vi "CompareZProfile2.vi"(5 "Z profile":dbl[](array[numeric])=[136.78057938360504, 136.0261652116635, 136.02991437413465, 127.00664231648236, 122.29049463775536, 113.645207456899, 109.8856960808644, 104.76567514371389, 100.83691644163049, 97.71438212515365, 93.93238486999432, 90.08654473167638, 87.00841340233623, 84.35416666666667, 81.7528515593838, 79.6393412331386, 83.05002287132794, 85.13533535994708, 91.11477171457702, 98.5078614332252, 103.77404656553082, 105.17571186727207, 109.49616358691677, 109.23224687693282, 112.95297246100046, 117.20435850121594, 115.42078946409929, 112.54404430067521, 102.6815824186669, 91.80857555867811, 81.43765852235101, 76.84419557315564, 77.3156658575995, 83.36916637000127, 89.63776385905682, 93.40653392326749, 107.04734731706081, 119.8811021895823, 151.17114676843892, 187.80852396310843, 214.26554708781225, 232.30872499497298, 224.32904818821265, 191.3640629515997, 147.3785829578186, 102.59016510146526, 80.02115124526546, 81.1632766895408, 95.07169339561545, 120.10465998090932, 137.718697100722, 143.98076644746772, 147.53366304165087, 141.65846157484788, 134.07428104411483, 129.81679576307346, 126.37067033940068, 121.24591602303097, 125.47090035098631, 122.74778342807349, 123.40827458303652, 123.34074109763333, 123.50642201559259, 120.7960259846455, 122.26527340257906] format="%.2f", 6 "Z LUT":dbl[][](array[numeric])=[[137.0, 137.0, 137.0, 130.0, 125.0, 119.0, 113.0, 108.0, 109.0, 114.0, 121.0, 127.0, 133.0, 139.0, 146.0, 153.0, 156.0, 151.0, 132.0, 100.0, 66.0, 46.0, 50.0, 72.0, 99.0, 119.0, 132.0, 138.0, 142.0, 146.0, 148.0, 149.0, 147.0, 143.0, 138.0, 133.0, 129.0, 128.0, 129.0, 130.0, 132.0, 134.0, 133.0, 132.0, 131.0, 130.0, 129.0, 129.0, 130.0, 130.0, 130.0, 130.0, 131.0, 131.0, 131.0, 131.0, 131.0, 131.0, 131.0, 131.0, 131.0, 131.0, 131.0, 131.0, 132.0], [135.0, 133.0, 130.0, 129.0, 130.0, 128.0, 119.0, 109.0, 101.0, 100.0, 104.0, 111.0, 119.0, 126.0, 134.0, 146.0, 162.0, 171.0, 164.0, 133.0, 88.0, 53.0, 42.0, 55.0, 80.0, 103.0, 124.0, 139.0, 151.0, 159.0, 160.0, 156.0, 150.0, 142.0, 135.0, 130.0, 128.0, 127.0, 130.0, 132.0, 132.0, 132.0, 131.0, 130.0, 130.0, 130.0, 130.0, 130.0, 131.0, 131.0, 129.0, 130.0, 131.0, 131.0, 132.0, 129.0, 131.0, 131.0, 132.0, 133.0, 133.0, 131.0, 131.0, 130.0, 132.0], [129.0, 128.0, 127.0, 127.0, 130.0, 129.0, 123.0, 114.0, 106.0, 98.0, 94.0, 95.0, 99.0, 107.0, 119.0, 142.0, 167.0, 186.0, 189.0, 163.0, 113.0, 63.0, 36.0, 37.0, 60.0, 87.0, 116.0, 139.0, 158.0, 168.0, 168.0, 161.0, 150.0, 141.0, 133.0, 129.0, 131.0, 130.0, 131.0, 132.0, 132.0, 132.0, 132.0, 131.0, 131.0, 130.0, 129.0, 130.0, 131.0, 130.0, 131.0, 131.0, 130.0, 130.0, 131.0, 130.0, 131.0, 132.0, 130.0, 131.0, 131.0, 131.0, 131.0, 131.0, 131.0], [129.0, 125.0, 125.0, 124.0, 127.0, 127.0, 124.0, 119.0, 111.0, 100.0, 91.0, 85.0, 85.0, 91.0, 103.0, 126.0, 159.0, 188.0, 200.0, 185.0, 140.0, 85.0, 43.0, 30.0, 42.0, 69.0, 103.0, 137.0, 163.0, 176.0, 176.0, 166.0, 154.0, 143.0, 136.0, 132.0, 131.0, 131.0, 131.0, 132.0, 132.0, 131.0, 132.0, 131.0, 131.0, 130.0, 130.0, 131.0, 130.0, 130.0, 130.0, 131.0, 130.0, 129.0, 129.0, 131.0, 130.0, 131.0, 130.0, 130.0, 130.0, 131.0, 131.0, 132.0, 132.0], [131.0, 126.0, 123.0, 121.0, 121.0, 123.0, 123.0, 120.0, 114.0, 104.0, 94.0, 85.0, 81.0, 82.0, 89.0, 106.0, 137.0, 174.0, 198.0, 197.0, 165.0, 115.0, 67.0, 39.0, 33.0, 49.0, 84.0, 126.0, 162.0, 181.0, 184.0, 175.0, 162.0, 150.0, 141.0, 135.0, 130.0, 129.0, 130.0, 132.0, 131.0, 130.0, 130.0, 131.0, 130.0, 131.0, 131.0, 132.0, 131.0, 130.0, 129.0, 130.0, 130.0, 130.0, 129.0, 130.0, 130.0, 131.0, 130.0, 131.0, 131.0, 131.0, 131.0, 131.0, 132.0], [132.0, 128.0, 122.0, 119.0, 117.0, 117.0, 118.0, 116.0, 112.0, 107.0, 100.0, 92.0, 87.0, 82.0, 82.0, 90.0, 113.0, 148.0, 179.0, 193.0, 181.0, 146.0, 102.0, 62.0, 37.0, 35.0, 61.0, 108.0, 152.0, 181.0, 190.0, 186.0, 174.0, 162.0, 148.0, 138.0, 130.0, 127.0, 127.0, 129.0, 130.0, 129.0, 129.0, 130.0, 129.0, 130.0, 131.0, 132.0, 132.0, 131.0, 130.0, 130.0, 131.0, 131.0, 131.0, 130.0, 130.0, 131.0, 132.0, 132.0, 132.0, 131.0, 131.0, 131.0, 132.0], [132.0, 128.0, 124.0, 120.0, 117.0, 114.0, 112.0, 111.0, 108.0, 106.0, 103.0, 99.0, 95.0, 90.0, 84.0, 84.0, 94.0, 120.0, 149.0, 174.0, 181.0, 168.0, 137.0, 95.0, 54.0, 33.0, 43.0, 83.0, 131.0, 169.0, 192.0, 197.0, 190.0, 176.0, 159.0, 144.0, 134.0, 127.0, 125.0, 125.0, 127.0, 128.0, 129.0, 130.0, 129.0, 130.0, 131.0, 132.0, 131.0, 131.0, 130.0, 130.0, 131.0, 131.0, 132.0, 131.0, 130.0, 131.0, 133.0, 133.0, 132.0, 131.0, 130.0, 131.0, 132.0], [131.0, 127.0, 125.0, 124.0, 119.0, 114.0, 110.0, 108.0, 105.0, 103.0, 101.0, 101.0, 100.0, 98.0, 94.0, 89.0, 87.0, 100.0, 119.0, 144.0, 164.0, 171.0, 161.0, 128.0, 82.0, 45.0, 34.0, 58.0, 102.0, 147.0, 185.0, 203.0, 205.0, 192.0, 174.0, 155.0, 139.0, 130.0, 124.0, 123.0, 125.0, 127.0, 128.0, 130.0, 130.0, 131.0, 132.0, 131.0, 130.0, 131.0, 130.0, 130.0, 129.0, 130.0, 131.0, 131.0, 131.0, 131.0, 132.0, 132.0, 132.0, 131.0, 132.0, 131.0, 132.0], [129.0, 125.0, 125.0, 125.0, 122.0, 117.0, 111.0, 108.0, 104.0, 101.0, 98.0, 98.0, 99.0, 102.0, 101.0, 98.0, 93.0, 94.0, 101.0, 115.0, 136.0, 156.0, 165.0, 151.0, 115.0, 70.0, 40.0, 42.0, 70.0, 116.0, 166.0, 200.0, 216.0, 209.0, 194.0, 172.0, 151.0, 134.0, 125.0, 122.0, 124.0, 126.0, 127.0, 129.0, 132.0, 132.0, 133.0, 131.0, 129.0, 131.0, 130.0, 130.0, 128.0, 129.0, 130.0, 130.0, 131.0, 131.0, 132.0, 131.0, 131.0, 130.0, 132.0, 131.0, 132.0], [129.0, 123.0, 125.0, 123.0, 122.0, 119.0, 114.0, 110.0, 105.0, 102.0, 97.0, 95.0, 94.0, 98.0, 102.0, 105.0, 102.0, 100.0, 97.0, 99.0, 111.0, 131.0, 151.0, 155.0, 138.0, 102.0, 61.0, 40.0, 46.0, 81.0, 135.0, 184.0, 216.0, 223.0, 216.0, 194.0, 169.0, 143.0, 128.0, 121.0, 121.0, 123.0, 126.0, 129.0, 133.0, 133.0, 134.0, 132.0, 131.0, 131.0, 130.0, 130.0, 129.0, 129.0, 129.0, 129.0, 130.0, 130.0, 131.0, 130.0, 129.0, 129.0, 131.0, 130.0, 133.0], [132.0, 123.0, 124.0, 122.0, 121.0, 119.0, 116.0, 112.0, 107.0, 103.0, 98.0, 93.0, 91.0, 91.0, 96.0, 103.0, 107.0, 109.0, 105.0, 100.0, 100.0, 109.0, 127.0, 143.0, 144.0, 126.0, 91.0, 56.0, 39.0, 53.0, 98.0, 153.0, 202.0, 227.0, 234.0, 217.0, 193.0, 161.0, 136.0, 121.0, 116.0, 118.0, 123.0, 128.0, 132.0, 133.0, 134.0, 133.0, 133.0, 131.0, 130.0, 130.0, 129.0, 130.0, 129.0, 129.0, 130.0, 129.0, 130.0, 129.0, 129.0, 129.0, 129.0, 130.0, 134.0], [135.0, 124.0, 125.0, 121.0, 119.0, 117.0, 114.0, 111.0, 107.0, 103.0, 98.0, 94.0, 90.0, 86.0, 88.0, 94.0, 104.0, 111.0, 114.0, 110.0, 105.0, 102.0, 108.0, 121.0, 132.0, 133.0, 115.0, 83.0, 52.0, 43.0, 65.0, 114.0, 172.0, 216.0, 240.0, 237.0, 219.0, 187.0, 153.0, 128.0, 114.0, 111.0, 116.0, 124.0, 129.0, 132.0, 134.0, 134.0, 133.0, 132.0, 131.0, 130.0, 130.0, 130.0, 130.0, 130.0, 131.0, 130.0, 130.0, 129.0, 130.0, 130.0, 130.0, 129.0, 133.0], [138.0, 127.0, 126.0, 123.0, 119.0, 116.0, 112.0, 108.0, 105.0, 102.0, 96.0, 94.0, 90.0, 85.0, 84.0, 86.0, 95.0, 106.0, 115.0, 119.0, 116.0, 110.0, 106.0, 107.0, 114.0, 122.0, 122.0, 105.0, 76.0, 53.0, 50.0, 77.0, 130.0, 187.0, 230.0, 246.0, 240.0, 217.0, 181.0, 145.0, 120.0, 108.0, 108.0, 116.0, 124.0, 130.0, 133.0, 134.0, 134.0, 132.0, 132.0, 131.0, 131.0, 131.0, 130.0, 132.0, 132.0, 131.0, 131.0, 130.0, 130.0, 131.0, 132.0, 131.0, 132.0], [139.0, 132.0, 128.0, 124.0, 120.0, 116.0, 111.0, 107.0, 102.0, 99.0, 94.0, 92.0, 89.0, 86.0, 84.0, 83.0, 88.0, 97.0, 107.0, 118.0, 124.0, 121.0, 116.0, 108.0, 105.0, 108.0, 112.0, 110.0, 96.0, 74.0, 57.0, 59.0, 91.0, 144.0, 201.0, 240.0, 250.0, 241.0, 213.0, 173.0, 136.0, 113.0, 104.0, 107.0, 116.0, 126.0, 132.0, 134.0, 135.0, 134.0, 132.0, 132.0, 131.0, 131.0, 131.0, 131.0, 132.0, 131.0, 132.0, 133.0, 131.0, 131.0, 132.0, 134.0, 133.0], [138.0, 135.0, 131.0, 125.0, 120.0, 117.0, 112.0, 108.0, 101.0, 97.0, 92.0, 90.0, 88.0, 85.0, 85.0, 84.0, 85.0, 91.0, 99.0, 109.0, 122.0, 126.0, 125.0, 119.0, 108.0, 102.0, 101.0, 101.0, 100.0, 90.0, 75.0, 62.0, 70.0, 103.0, 157.0, 211.0, 245.0, 252.0, 240.0, 209.0, 164.0, 128.0, 108.0, 101.0, 107.0, 118.0, 128.0, 134.0, 136.0, 136.0, 134.0, 133.0, 131.0, 131.0, 131.0, 131.0, 131.0, 131.0, 131.0, 132.0, 132.0, 132.0, 132.0, 134.0, 134.0], [138.0, 136.0, 132.0, 128.0, 121.0, 117.0, 112.0, 108.0, 103.0, 98.0, 92.0, 89.0, 87.0, 86.0, 85.0, 86.0, 88.0, 90.0, 96.0, 101.0, 113.0, 122.0, 128.0, 127.0, 119.0, 107.0, 98.0, 93.0, 93.0, 93.0, 87.0, 76.0, 70.0, 80.0, 116.0, 168.0, 218.0, 248.0, 252.0, 238.0, 203.0, 157.0, 122.0, 103.0, 100.0, 110.0, 121.0, 132.0, 137.0, 138.0, 138.0, 135.0, 133.0, 131.0, 130.0, 130.0, 131.0, 130.0, 130.0, 131.0, 131.0, 133.0, 132.0, 134.0, 134.0], [137.0, 135.0, 133.0, 127.0, 122.0, 117.0, 113.0, 107.0, 102.0, 99.0, 94.0, 90.0, 87.0, 85.0, 86.0, 86.0, 90.0, 93.0, 96.0, 99.0, 106.0, 114.0, 122.0, 128.0, 126.0, 117.0, 104.0, 93.0, 87.0, 87.0, 89.0, 86.0, 80.0, 78.0, 92.0, 128.0, 176.0, 224.0, 248.0, 251.0, 234.0, 197.0, 151.0, 116.0, 99.0, 102.0, 112.0, 127.0, 137.0, 140.0, 141.0, 139.0, 136.0, 132.0, 130.0, 128.0, 130.0, 129.0, 129.0, 130.0, 130.0, 131.0, 132.0, 133.0, 133.0], [136.0, 134.0, 133.0, 127.0, 121.0, 116.0, 112.0, 107.0, 102.0, 98.0, 95.0, 91.0, 88.0, 85.0, 85.0, 86.0, 90.0, 94.0, 98.0, 101.0, 104.0, 108.0, 115.0, 122.0, 125.0, 124.0, 114.0, 100.0, 88.0, 82.0, 84.0, 87.0, 89.0, 87.0, 90.0, 106.0, 138.0, 183.0, 226.0, 248.0, 249.0, 229.0, 189.0, 143.0, 109.0, 97.0, 102.0, 117.0, 132.0, 141.0, 145.0, 144.0, 140.0, 136.0, 133.0, 128.0, 128.0, 129.0, 128.0, 130.0, 130.0, 130.0, 130.0, 131.0, 132.0], [135.0, 134.0, 133.0, 127.0, 121.0, 114.0, 111.0, 107.0, 102.0, 98.0, 94.0, 92.0, 89.0, 87.0, 85.0, 85.0, 88.0, 93.0, 98.0, 103.0, 106.0, 108.0, 111.0, 115.0, 119.0, 122.0, 119.0, 110.0, 97.0, 85.0, 80.0, 83.0, 89.0, 93.0, 97.0, 104.0, 120.0, 148.0, 189.0, 225.0, 246.0, 244.0, 221.0, 179.0, 134.0, 103.0, 94.0, 104.0, 121.0, 137.0, 146.0, 149.0, 146.0, 141.0, 136.0, 131.0, 128.0, 127.0, 128.0, 130.0, 131.0, 130.0, 131.0, 130.0, 130.0], [132.0, 132.0, 133.0, 128.0, 122.0, 115.0, 109.0, 106.0, 101.0, 98.0, 95.0, 92.0, 89.0, 87.0, 85.0, 84.0, 85.0, 90.0, 96.0, 102.0, 106.0, 110.0, 112.0, 113.0, 115.0, 118.0, 118.0, 114.0, 107.0, 95.0, 85.0, 81.0, 84.0, 92.0, 101.0, 109.0, 119.0, 134.0, 160.0, 193.0, 224.0, 240.0, 236.0, 210.0, 169.0, 125.0, 97.0, 93.0, 105.0, 125.0, 142.0, 151.0, 152.0, 148.0, 141.0, 135.0, 130.0, 127.0, 127.0, 129.0, 130.0, 131.0, 132.0, 131.0, 129.0], [131.0, 131.0, 131.0, 129.0, 123.0, 116.0, 110.0, 105.0, 101.0, 98.0, 95.0, 92.0, 89.0, 86.0, 84.0, 84.0, 84.0, 87.0, 92.0, 98.0, 104.0, 109.0, 113.0, 114.0, 116.0, 115.0, 116.0, 114.0, 111.0, 103.0, 94.0, 86.0, 82.0, 87.0, 98.0, 110.0, 123.0, 134.0, 148.0, 169.0, 196.0, 220.0, 231.0, 224.0, 198.0, 157.0, 116.0, 94.0, 92.0, 107.0, 129.0, 147.0, 155.0, 155.0, 148.0, 141.0, 134.0, 128.0, 127.0, 128.0, 129.0, 131.0, 132.0, 133.0, 130.0], [129.0, 129.0, 130.0, 128.0, 123.0, 117.0, 111.0, 106.0, 101.0, 98.0, 95.0, 93.0, 90.0, 86.0, 84.0, 82.0, 83.0, 85.0, 89.0, 95.0, 101.0, 107.0, 111.0, 115.0, 118.0, 117.0, 116.0, 114.0, 110.0, 107.0, 101.0, 93.0, 86.0, 85.0, 91.0, 104.0, 121.0, 135.0, 148.0, 161.0, 178.0, 197.0, 213.0, 220.0, 211.0, 185.0, 145.0, 111.0, 92.0, 94.0, 111.0, 134.0, 151.0, 159.0, 157.0, 150.0, 140.0, 133.0, 128.0, 127.0, 128.0, 130.0, 131.0, 133.0, 132.0], [128.0, 127.0, 128.0, 126.0, 123.0, 117.0, 112.0, 107.0, 102.0, 98.0, 96.0, 93.0, 92.0, 88.0, 84.0, 83.0, 82.0, 84.0, 87.0, 93.0, 99.0, 105.0, 110.0, 114.0, 118.0, 119.0, 118.0, 115.0, 111.0, 107.0, 103.0, 98.0, 92.0, 88.0, 88.0, 96.0, 112.0, 129.0, 146.0, 161.0, 172.0, 185.0, 195.0, 205.0, 206.0, 197.0, 170.0, 138.0, 108.0, 93.0, 97.0, 116.0, 138.0, 156.0, 162.0, 159.0, 151.0, 141.0, 132.0, 128.0, 127.0, 128.0, 130.0, 132.0, 132.0], [127.0, 125.0, 126.0, 124.0, 121.0, 117.0, 112.0, 107.0, 102.0, 98.0, 96.0, 95.0, 92.0, 91.0, 86.0, 84.0, 83.0, 83.0, 86.0, 91.0, 97.0, 103.0, 109.0, 113.0, 117.0, 119.0, 120.0, 117.0, 113.0, 109.0, 102.0, 99.0, 95.0, 92.0, 90.0, 93.0, 103.0, 118.0, 136.0, 157.0, 171.0, 182.0, 189.0, 194.0, 196.0, 194.0, 182.0, 159.0, 131.0, 105.0, 96.0, 101.0, 120.0, 143.0, 159.0, 165.0, 162.0, 152.0, 141.0, 132.0, 128.0, 126.0, 127.0, 131.0, 132.0], [129.0, 124.0, 124.0, 122.0, 119.0, 116.0, 111.0, 107.0, 101.0, 97.0, 94.0, 93.0, 93.0, 91.0, 90.0, 86.0, 85.0, 85.0, 86.0, 90.0, 96.0, 101.0, 108.0, 113.0, 116.0, 120.0, 119.0, 119.0, 114.0, 111.0, 105.0, 100.0, 96.0, 92.0, 93.0, 93.0, 99.0, 109.0, 125.0, 145.0, 164.0, 179.0, 188.0, 192.0, 191.0, 187.0, 182.0, 167.0, 149.0, 124.0, 106.0, 97.0, 105.0, 125.0, 147.0, 162.0, 168.0, 163.0, 153.0, 142.0, 132.0, 127.0, 125.0, 127.0, 132.0], [131.0, 126.0, 125.0, 122.0, 119.0, 115.0, 111.0, 105.0, 101.0, 95.0, 93.0, 90.0, 91.0, 91.0, 90.0, 90.0, 87.0, 86.0, 87.0, 89.0, 96.0, 100.0, 106.0, 112.0, 115.0, 119.0, 119.0, 119.0, 116.0, 112.0, 107.0, 103.0, 98.0, 94.0, 95.0, 95.0, 98.0, 106.0, 117.0, 134.0, 153.0, 170.0, 185.0, 192.0, 193.0, 186.0, 180.0, 168.0, 156.0, 138.0, 118.0, 104.0, 98.0, 109.0, 128.0, 150.0, 166.0, 171.0, 165.0, 154.0, 141.0, 132.0, 126.0, 125.0, 129.0], [130.0, 128.0, 127.0, 124.0, 120.0, 115.0, 110.0, 105.0, 100.0, 95.0, 91.0, 89.0, 88.0, 90.0, 90.0, 91.0, 89.0, 88.0, 88.0, 89.0, 94.0, 98.0, 104.0, 111.0, 114.0, 118.0, 118.0, 119.0, 117.0, 115.0, 109.0, 106.0, 101.0, 97.0, 96.0, 97.0, 100.0, 106.0, 115.0, 127.0, 142.0, 160.0, 177.0, 189.0, 194.0, 191.0, 183.0, 170.0, 158.0, 143.0, 127.0, 113.0, 101.0, 101.0, 111.0, 131.0, 153.0, 168.0, 172.0, 167.0, 154.0, 141.0, 131.0, 126.0, 125.0], [127.0, 127.0, 127.0, 124.0, 121.0, 116.0, 111.0, 106.0, 100.0, 95.0, 91.0, 88.0, 86.0, 88.0, 89.0, 91.0, 91.0, 91.0, 89.0, 89.0, 93.0, 96.0, 102.0, 108.0, 113.0, 118.0, 119.0, 119.0, 118.0, 116.0, 112.0, 108.0, 104.0, 100.0, 97.0, 98.0, 100.0, 105.0, 114.0, 124.0, 136.0, 151.0, 166.0, 181.0, 191.0, 193.0, 189.0, 176.0, 162.0, 146.0, 132.0, 120.0, 108.0, 103.0, 104.0, 115.0, 134.0, 154.0, 168.0, 172.0, 166.0, 153.0, 141.0, 131.0, 126.0], [127.0, 126.0, 124.0, 122.0, 119.0, 116.0, 111.0, 107.0, 102.0, 96.0, 92.0, 89.0, 86.0, 85.0, 87.0, 89.0, 91.0, 92.0, 90.0, 90.0, 92.0, 94.0, 99.0, 105.0, 111.0, 117.0, 119.0, 120.0, 120.0, 118.0, 115.0, 111.0, 106.0, 102.0, 99.0, 98.0, 98.0, 103.0, 111.0, 121.0, 132.0, 145.0, 158.0, 172.0, 183.0, 190.0, 191.0, 184.0, 170.0, 153.0, 136.0, 123.0, 113.0, 108.0, 106.0, 111.0, 121.0, 138.0, 154.0, 165.0, 169.0, 163.0, 153.0, 141.0, 132.0], [137.0, 125.0, 123.0, 123.0, 120.0, 117.0, 112.0, 107.0, 101.0, 96.0, 91.0, 87.0, 85.0, 84.0, 85.0, 87.0, 89.0, 91.0, 93.0, 93.0, 94.0, 95.0, 99.0, 104.0, 109.0, 114.0, 118.0, 120.0, 120.0, 119.0, 116.0, 111.0, 108.0, 104.0, 101.0, 99.0, 99.0, 102.0, 108.0, 117.0, 128.0, 140.0, 153.0, 165.0, 176.0, 184.0, 188.0, 185.0, 178.0, 163.0, 145.0, 129.0, 116.0, 109.0, 107.0, 108.0, 115.0, 126.0, 140.0, 154.0, 166.0, 167.0, 162.0, 152.0, 141.0]], 7 "error in 2":errorcluster, 8 "Cutoff R(bins)":i32) -> (0 "error out3":errorcluster, 2 "min index (indices)":dbl=18.32291011013138 format="%.2f")   [LabVIEW 2011, in "OfflineTracker.lvlib"]
uses:
  OfflineTracker.lvlib
  <vilib>/Analysis/2dsp.llb/Inverse Complex FFT.vi
  <vilib>/Analysis/2dsp.llb/Real FFT.vi
  <vilib>/Analysis/NI_AALPro.lvlib
panel:
  out "Profiles":dbl[][](graph)
  out "difference":dbl[](graph)=[-969082.0972984378, -967037.7722979455, -964804.9246087972, -962668.7351843655, -961215.9984278528, -960301.9664475948, -959117.4038459591, -957399.5427407083, -956060.421729733, -954513.8410193664, -953987.4056031316, -954132.6257660121, -958177.4561058765, -965201.3884337995, -974167.5629561953, -987609.8930113036, -1000735.5039044532, -1011765.2445241701, -1017546.197679587, -1016304.9716130408, -1008125.9686854713, -997567.0878852411, -987672.1264481557, -980349.3211130741, -974093.1395069708, -968786.8162099749, -963613.5362654983, -958109.0158232427, -952208.5596050965, -948737.7610081622]
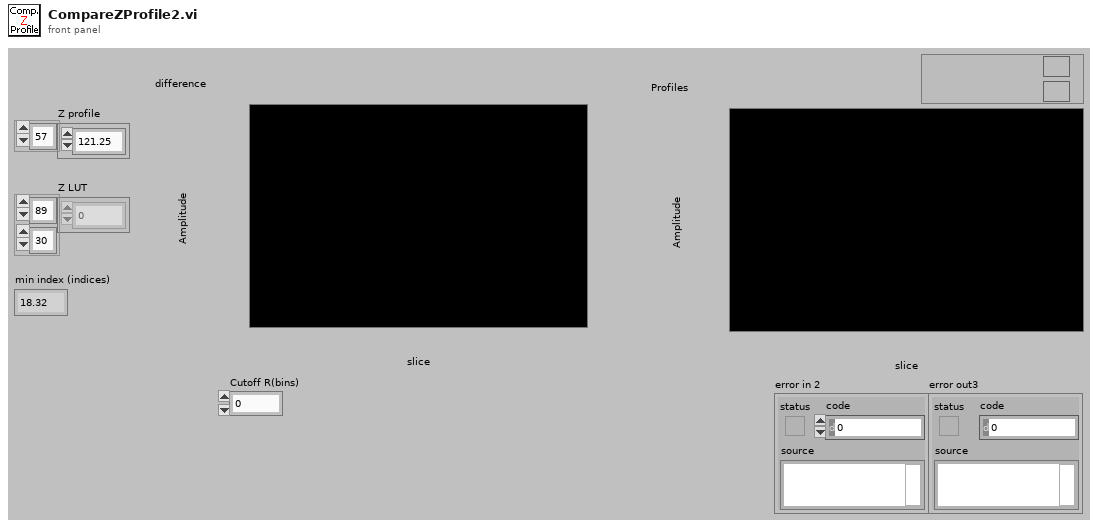
[diagram p1: front panel]
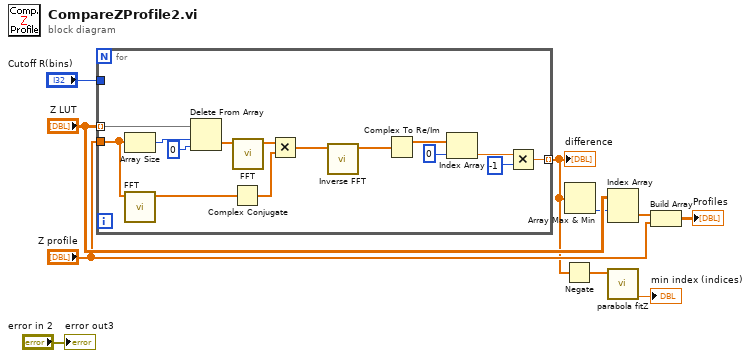
[diagram p0: block diagram]
diagram:
  n1 = for {
    tunnel: "Z LUT" -> [w21] mode=indexing
    tunnel: [w25] -> w3 mode=indexing
    tunnel: "Z profile" -> [w24]
    tunnel: "Cutoff R(bins)" -> [_]
    n2 = Array Size(array=w24) -> (size(s)=w23:i32)
    n3 = call-poly <vilib>:"FFT.vi"("X"=w24) -> ("FFT {X}"=w19:cdb[])  [unwired: 2 in, 8 out]
    n4 = Delete From Array(array=w21, length=w23, index=0) -> (deleted portion=w20:dbl[])  [unwired: 1 out]
    n5 = Complex Conjugate(1:w19) -> (0:w17:cdb[])
    n6 = call-poly <vilib>:"FFT.vi"("X"=w20) -> ("FFT {X}"=w18:cdb[])  [unwired: 2 in, 8 out]
    n7 = Multiply(x=w18, y=w17) -> (x*y=w16:cdb[])
    n8 = call-poly <vilib>:"Inverse FFT.vi"("FFT {X}"=w16) -> ("X"=w15:cdb[])  [unwired: 1 in, 9 out]
    n9 = Complex To Re/Im(x + iy=w15) -> (x=w14:dbl[])  [unwired: 1 out]
    n10 = Index Array(array=w14, index=0) -> (element=w12:dbl)
    n11 = Multiply(x=w12, y=-1) -> (x*y=w25:dbl)
  }
  "difference" <- w3
  n12 = Negate(x=w3) -> (-x=w2:dbl[])
  n13 = Array Max & Min(array=w3) -> (min index (indices)=w8:i32)  [unwired: 3 out]
  n14 = Index Array(array="Z LUT", index (row)=w8) -> (element=w7:dbl[])  [unwired: 1 in]
  n15 = call "parabola fitZ.vi"("radial profile"=w2) -> ("Y focus"=→"min index (indices)":dbl)  [unwired: 7 in]
  n16 = Build Array(w7, "Z profile") -> (→"Profiles":dbl[][])
  "error out3" <- "error in 2"
